vi "initialise_boxes.vi"(10 "Dataset Directory":path=path "C:/Users/Naomi Tan/Documents/Gillette/ML/STIR_ML_dev/LabView/original_images/IMG_6155.JPG", 11 "Image Directory":path=path "C:/Users/Naomi Tan/Documents/Gillette/ML/STIR_ML_dev/LabView/original_images/IMG_6155.JPG") -> (0 "Number of Points":i32, 1 "Initial Bounding Boxes":T2(array[cluster]), 2 "Initial Data":string[][](array[string])=[["file_name", "x_min", "y_min", "x_max", "y_max", "class"]], 3 "Image Out":T1, 4 "Existing Filename":string)   [LabVIEW 2017]
uses:
  <vilib>/vision/Image Controls.llb/IMAQ Image.ctl
  <vilib>/Utility/file.llb/Read Delimited Spreadsheet (string).vi
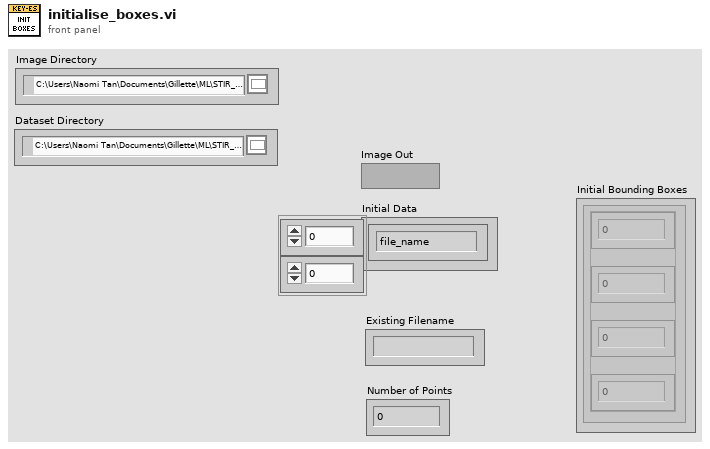
[diagram p1: front panel]
types:
  T1 = typedef "IMAQ Image.ctl" = refnum<image>
  T2 = cluster{"[0]":i32, "[1]":i32, "[2]":i32, "[3]":i32}[]
  T3 = typedef "Image Type" = u32
  T4 = cluster{"[0]":i32, "[1]":i32, "[2]":i32, "[3]":i32}
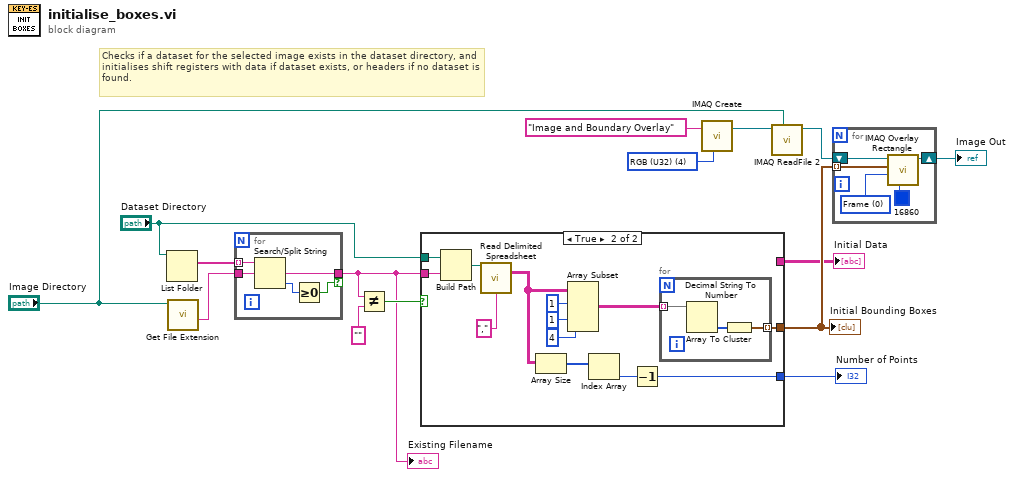
[diagram p0: block diagram]
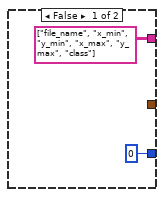
[diagram p2: hidden frame]
diagram:
  w9 = T3 4 items=["Grayscale (U8)", "Grayscale (I16)", "Grayscale (SGL)", "Complex (CSG)", "RGB (U32)", "HSL (U32)", "RGB (U64)", "Grayscale (U16)"] ("Image Type")
  # "Checks if a dataset for the selected image exists in the dataset directory, and initialises shift registers with data if dataset exists, or headers if no dataset is found."
  n1 = List Folder(path="Dataset Directory") -> (filenames=w15:string[])  [unwired: 3 in, 3 out]
  n2 = call <vilib>:"Get File Extension.vi"("file"="Image Directory") -> ("filename without extension"=w14:string)  [unwired: 6 in, 4 out]
  n3 = for {
    tunnel: w15 -> [w19] mode=indexing
    tunnel: w14 -> [w20]
    tunnel: [w18] -> w11 if=w16
    n4 = Search/Split String(string=w19, search string/char (-)=w20) -> (match + rest of string=w18:string, offset of match=w17:i32)  [unwired: 1 in, 1 out]
    n5 = Greater Or Equal To 0?(x=w17) -> (x >= 0?=w16:bool)
  }
  "Existing Filename" <- w11
  n6 = Not Equal?(x=w11, y="" ("delimiter (\\t)")) -> (x != y?=w13:bool)
  n7 = case shown="True" w13 {
    tunnel: w11 -> [_ w34]
    tunnel: "Dataset Directory" -> [_ w33]
    tunnel: [_ w27] -> w10
    tunnel: [string[][] [["file_name", "x_min", "y_min", "x_max", "y_max", "class"]] _] -> w3
    tunnel: [0 w23] -> w1
    frame False {
    }
    frame True {
      n8 = Build Path(base path=w33, name or relative path=w34) -> (appended path=w32:path)
      n9 = call-poly <vilib>:"Read Delimited Spreadsheet.vi"("file path (dialog if empty)"=w32, "delimiter (\\t)"="," ("delimiter (\\t)")) -> ("all rows"=w26:string[][])  [unwired: 8 in, 5 out]
      n10 = Array Size(array=w26) -> (size(s)=w25:i32[])
      n11 = Array Subset(array=w26, index (row)=1 ("index"), index (col)=1 ("index"), length (col)=4 ("index")) -> (w28:string[][])  [unwired: 1 in]
      n12 = Index Array(array=w25) -> (element=w24:i32)  [unwired: 1 in]
      n13 = Decrement(x=w24) -> (x-1=w23:i32)
      n14 = for {
        tunnel: w28 -> [w38] mode=indexing
        tunnel: [w36] -> w27 mode=indexing
        n15 = Decimal String To Number(string=w38) -> (number=w37:i32[])  [unwired: 2 in, 1 out]
        n16 = Array To Cluster(array=w37) -> (cluster=w36:T4)
      }
    }
  }
  "Initial Bounding Boxes" <- w10
  "Initial Data" <- w3
  "Number of Points" <- w1
  n17 = call "IMAQ Create"("Image Name"="Image and Boundary Overlay", "Image Type"=w9) -> ("New Image"=w8:T1)  [unwired: 3 in, 1 out]
  n18 = call "IMAQ ReadFile 2"("File Path"="Image Directory", "Image"=w8) -> ("Image Out"=w7:T1)  [unwired: 5 in, 4 out]
  n19 = for {
    tunnel: w10 -> [w41] mode=indexing
    shift-right: [w42] -> w5
    shift-left: w7 -> [w43]
    w40 = u32 0 items=["Frame", "Fill"] ("Drawing Mode (Frame)")
    n20 = call "IMAQ Overlay Rectangle"("Color"=u32 16860, "Drawing Mode (Frame)"=w40, "Rectangle"=w41, "Image"=w43) -> ("Image Out"=w42:T1)  [unwired: 6 in, 1 out]
  }
  "Image Out" <- w5
